vi "Reference Model Joystick.vi"(1 "dt":dbl=0.2, 2 "Reset Array":bool[](array[boolean])=[FALSE, FALSE, FALSE, FALSE, FALSE, FALSE], 3 "Reset":bool, 7 "Reference Joystick":dbl[](array[numeric])=[0.0, 0.0, 0.0, 0.0, 0.0, 0.0], 11 "Error In":errorcluster, 12 "Omega":dbl[](array[numeric])=[0.8, 0.8, 0.8, 0.8, 0.8, 0.8], 13 "Delta":dbl[](array[numeric])=[1.0, 1.0, 1.0, 1.0, 1.0, 1.0]) -> (6 "nu_desired":dbl[](array[numeric]), 15 "Error Out":errorcluster)   [LabVIEW 2014]
uses:
  <vilib>/imath/engines/lvmath2/RunTimeEngine/RangeToken/NIMS_Range_R2 - Integer.vi
  <instcachedir>/0/NIMS_Range_R2 - Integer_2D1304BAF97744E0A293025746CBADFC.lvgen/NIMS_Range_R2 - Integer_2D1304BAF97744E0A293025746CBADFC_000.vi
  <vilib>/imath/engines/lvmath2/RunTimeEngine/CommandStatement/MC_CommandStatement_break.vi
  <vilib>/imath/engines/lvmath2/RunTimeEngine/IndexRead/NIMS V(S).vi
  <instcachedir>/0/NIMS V(S)_0488751826AF41519A22953C041130DC.lvgen/NIMS V(S)_0488751826AF41519A22953C041130DC_000.vi
  <vilib>/imath/engines/lvmath2/RunTimeEngine/IndexReplace/NIMS V(S)=S.vi
  <instcachedir>/0/NIMS V(S)=S_2D52C4EC15D8415E870AEE69FB516CCA.lvgen/NIMS V(S)=S_2D52C4EC15D8415E870AEE69FB516CCA_000.vi
  <vilib>/imath/engines/lvmath2/RunTimeEngine/ErrorHandling/NIMS_Create Error From Enums.vi
  <vilib>/imath/engines/lvmath2/RunTimeEngine/NodeEndStatement/NIMS_NodeEndStatement_Output.vi
  <instcachedir>/0/NIMS_NodeEndStatement_Output_53EC0D466D134D7ABD903AC30B43404B.lvgen/NIMS_NodeEndStatement_Output_53EC0D466D134D7ABD903AC30B43404B_005.vi
  <vilib>/imath/engines/lvmath2/RunTimeEngine/ErrorHandling/NIMS_Finalize Error.vi
  Library/Integrator/Integrator trapez vector.vi
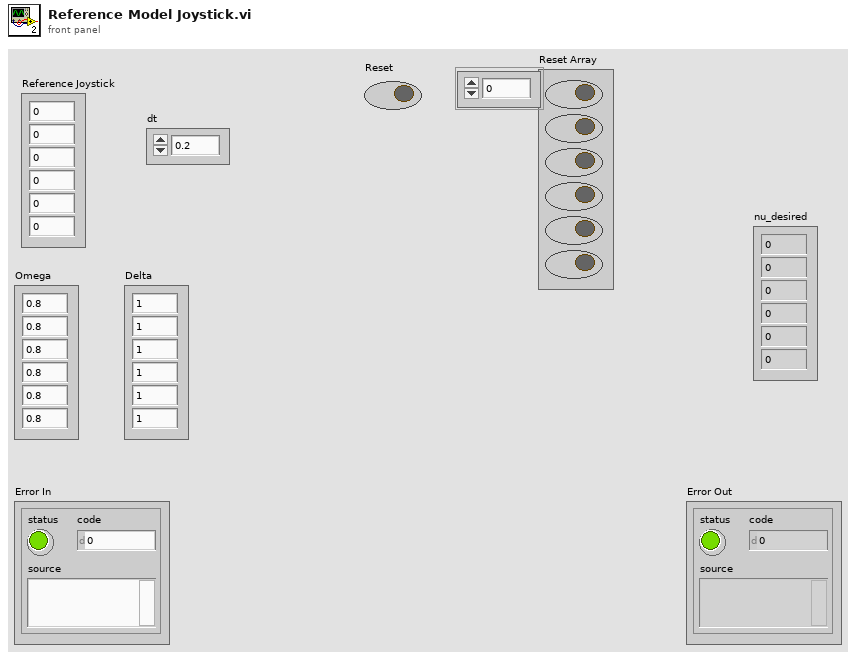
[diagram p1: front panel]
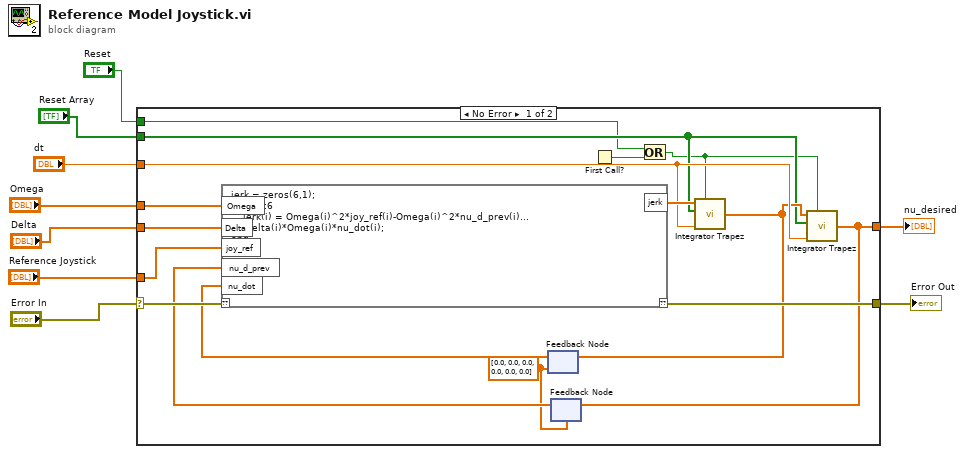
[diagram p0: block diagram]
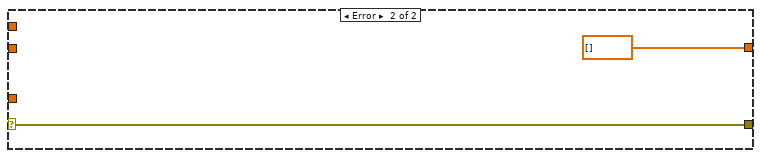
[diagram p2: hidden frame]
diagram:
  n1 = case shown="No Error" "Error In" {
    selector: "Error In" -> [w22 w154]
    tunnel: "Omega" -> [w25 _]
    tunnel: "Delta" -> [w24 _]
    tunnel: "Reference Joystick" -> [w23 _]
    tunnel: "dt" -> [w19 _]
    tunnel: [w14 dbl[] []] -> w4
    tunnel: [w17 w154] -> w3
    tunnel: "Reset Array" -> [w13 _]
    tunnel: "Reset" -> [w10 _]
    frame No Error {
      w16 = dbl[] [0.0, 0.0, 0.0, 0.0, 0.0, 0.0]
      n2 = feedback #1(w16) -> (w20:dbl[])
      n3 = feedback #2(w16) -> (w18:dbl[])
      n4 = mathscript code="jerk = zeros(6,1);\nfor i=1:6\n    jerk(i) = Omega(i)^2*joy_ref(i)-Omega(i)^2*nu_d_prev(i)...\n-2*Delta(i)*Omega(i)*nu_dot(i);\nend"("??"=w22, "Omega"=w25, "Delta"=w24, "joy_ref"=w23, "nu_d_prev"=w18, "nu_dot"=w20) -> ("??"=w17:errorcluster, "jerk"=w21:dbl[])
      n5 = First Call?() -> (First Call?: T/F=w12:bool)
      n6 = Or(x=w10, y=w12) -> (x .or. y?=w11:bool)
      n7 = call-poly "Integrator Trapez.vi"("Reset"=w11, "dt"=w19, "Reset Array"=w13, "Input"=w21) -> ("Output"=w15:dbl[])  [unwired: 2 in]
      n8 = feedback-in #1(w15) -> ()
      n9 = call-poly "Integrator Trapez.vi"("Reset"=w11, "dt"=w19, "Reset Array"=w13, "Input"=w15) -> ("Output"=w14:dbl[])  [unwired: 2 in]
      n10 = feedback-in #2(w14) -> ()
    }
    frame Error {
    }
  }
  "nu_desired" <- w4
  "Error Out" <- w3
